vi "FlushSink.vi"(8 "error in (no error)":errorcluster, 11 "RelayAppender in":refnum<class "RelayAppender.lvclass">) -> (0 "error out":errorcluster, 3 "RelayAppender out":refnum<class "RelayAppender.lvclass">)   [LabVIEW 2026, in "Lumberjack.lvlib" / "RelayAppender.lvclass"]
uses:
  RelayAppender.lvclass
  RelayAppender.lvclass/RelayAppender.ctl
  Appender.lvclass/Appender.lvclass
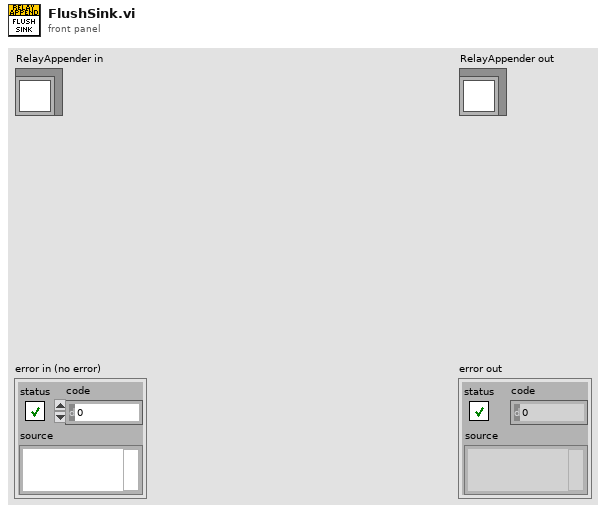
[diagram p1: front panel]
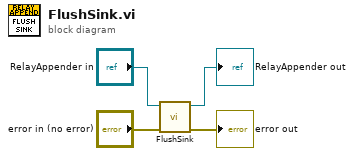
[diagram p0: block diagram]
diagram:
  n1 = call-parent "FlushSink.vi"("error in (no error)"="error in (no error)", "Appender in"="RelayAppender in") -> ("error out"=→"error out":errorcluster, "Appender out"=→"RelayAppender out":refnum<class "RelayAppender.lvclass">)  [unwired: 8 in]
